vi "Add DAQmx Channels.vi"(9 "Tasks":refnum<k21>[](array[refnum]), 10 "Spares":string[](array[string]), 11 "Sensor List Class in":T1) -> (3 "Sensor List Class out":T1)   [LabVIEW 2013, in "Sensors Page X.xctl"]
uses:
  XControls/Sensors Page X.xctl
  Data Access Objects/Sensors/Sensor List Class.lvclass
  XControls/Sensors Page Data.ctl
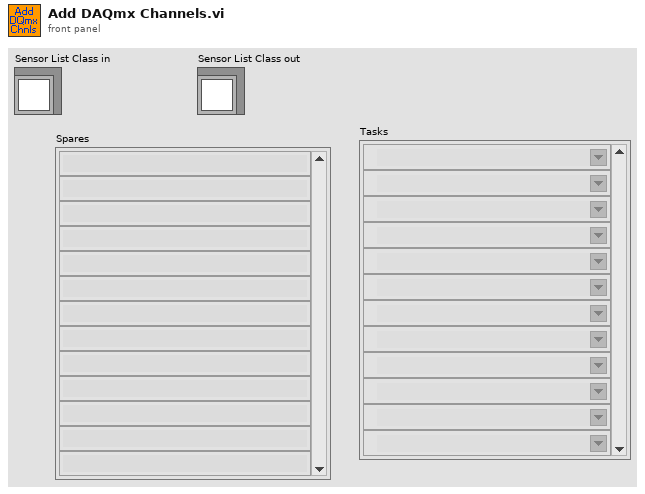
[diagram p1: front panel]
types:
  T1 = typedef "Sensors Page X.xctl/Sensors Page Data.ctl" = refnum<class "Sensor List Class.lvclass">
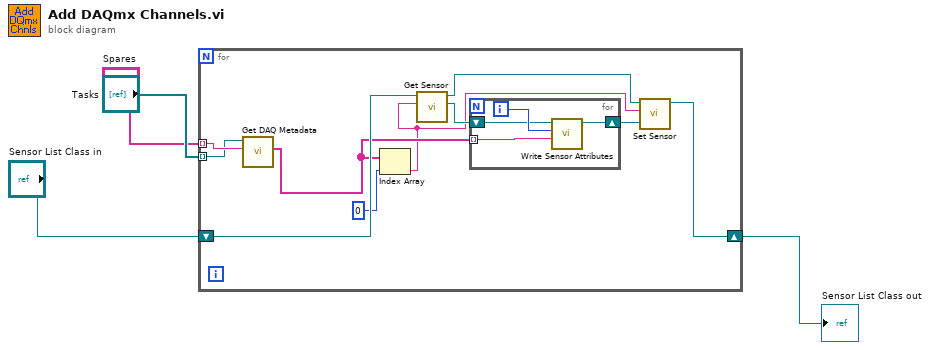
[diagram p0: block diagram]
diagram:
  n1 = for {
    shift-right: [w13] -> w1
    shift-left: "Sensor List Class in" -> [w14]
    tunnel: "Spares" -> [w12] mode=indexing
    tunnel: "Tasks" -> [w11] mode=indexing
    n2 = call "Get DAQ Metadata.vi"("Channel"=w12, "Task"=w11) -> ("Metadata"=w10:string[])  [unwired: 9 in]
    n3 = Index Array(array=w10, index=0) -> (element=w5:string)
    n4 = call "Get Sensor.vi"("Name"=w5, "Sensor List Class in"=w14) -> ("Sensor DAO Out"=w8:refnum<class "Sensor DAO Class.lvclass">, "Sensor List Class out"=w6:T1)  [unwired: 7 in, 1 out]
    n5 = for {
      tunnel: w10 -> [w18] mode=indexing
      shift-right: [w15] -> w7
      shift-left: w8 -> [w16]
      i -> [w17]
      n6 = call "Write Sensor Attributes.vi"("New"=w18, 10:w17, "Sensor DAO Class in"=w16) -> ("Sensor DAO Class out"=w15:refnum<class "Sensor DAO Class.lvclass">)  [unwired: 8 in]
    }
    n7 = call "Set Sensor.vi"("Sensor DAO In"=w7, "Name"=w5, "Sensor List Class in"=w6) -> ("Sensor List Class out"=w13:T1)  [unwired: 7 in, 1 out]
  }
  "Sensor List Class out" <- w1
